vi "Statusword_ModeSpecific_PositionProfile.vi"(11 "StatusWord In":u16 format="%08b") -> (0 "Set Point Reached?":bool, 1 "Following Error":bool, 2 "Set Point Acknowledged":bool, 3 "StatusWord Out":u16 format="%08b")   [LabVIEW 2017, in "WordManipulationLibrary.lvlib"]
uses:
  WordManipulationLibrary.lvlib
  Bit Manipulation.lvlib
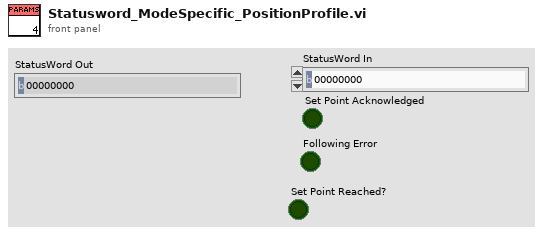
[diagram p1: front panel]
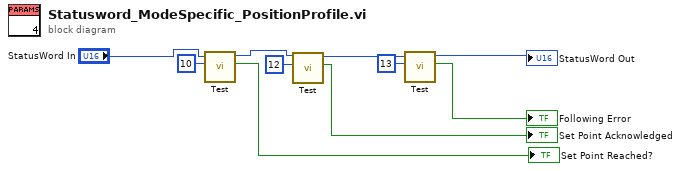
[diagram p0: block diagram]
diagram:
  n1 = call "Test.vi"("Bit to test"=u8 10, "Data_In"="StatusWord In") -> ("bit value"=→"Set Point Reached?":bool, "Data_Out"=w2:u16)  [unwired: 8 in]
  n2 = call "Test.vi"("Bit to test"=u8 12, "Data_In"=w2) -> ("bit value"=→"Set Point Acknowledged":bool, "Data_Out"=w8:u16)  [unwired: 8 in]
  n3 = call "Test.vi"("Bit to test"=u8 13, "Data_In"=w8) -> ("bit value"=→"Following Error":bool, "Data_Out"=→"StatusWord Out":u16)  [unwired: 8 in]
